vi "Gather Mean.vi"(10 "JSON Array":refnum<class "JSON Array.lvclass">, 11 "Statistics in":refnum<class "JSON Value.lvclass">) -> (3 "Statistics out":refnum<class "JSON Value.lvclass">)   [LabVIEW 2020, in "Library Commun.lvlib" / "JSON Array.lvclass"]
uses:
  JSON Array.lvclass
  JSON Value/JSON Value.lvclass
  C:/Users/ngarcin/OneDrive - Altyor/Standard TB/Class/JSON API/JSON Value/JSON Value.lvclass
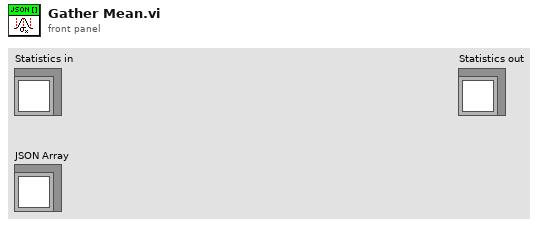
[diagram p1: front panel]
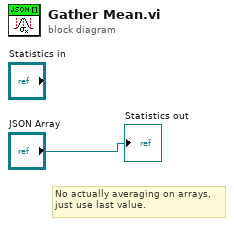
[diagram p0: block diagram]
diagram:
  # "No actually averaging on arrays,\njust use last value."
  "Statistics out" <- "JSON Array"
